vi "Write Elevator Direction.vi"(8 "error in (no error)":errorcluster, 10 "Elevator Direction":T1, 11 "Display Console in":refnum<class "Display Console.lvclass">) -> (0 "error out":errorcluster, 3 "Display Console out":refnum<class "Display Console.lvclass">)   [LabVIEW 2019, in "Display Console Actor.lvlib" / "Display Console.lvclass"]
uses:
  Display Console.lvclass
  Elevator Direction.ctl
  Display Console.lvclass/Display Console.ctl
  Abstract Display Console Actor/Abstract Display Console Actor/Abstract Display Console.lvclass
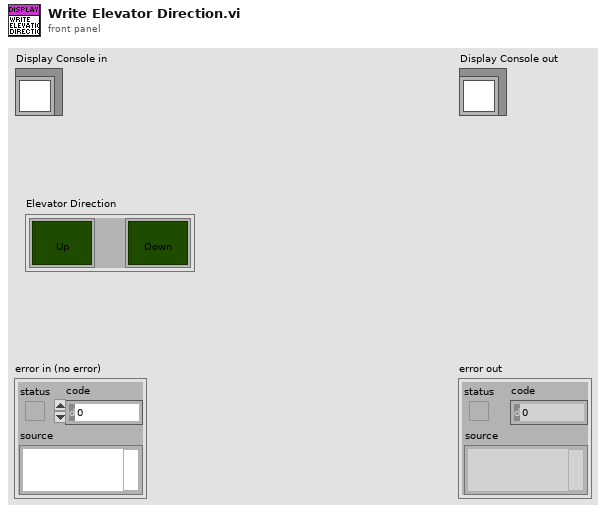
[diagram p1: front panel]
types:
  T1 = typedef "Display Console Actor.lvlib/Display Console.lvclass/Elevator Direction.ctl" = cluster{"Up":bool, "Down":bool}
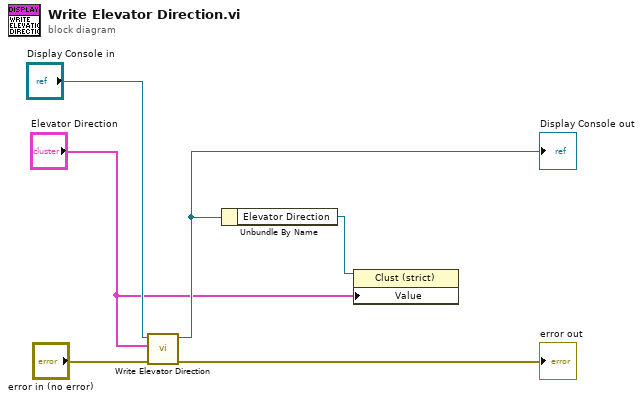
[diagram p0: block diagram]
diagram:
  n1 = call-parent "Write Elevator Direction.vi"("error in (no error)"="error in (no error)", "Elevator Direction"="Elevator Direction", "Abstract Display Console in"="Display Console in") -> ("error out"=→"error out":errorcluster, "Abstract Display Console out"=w3:refnum<class "Display Console.lvclass">)  [unwired: 7 in]
  "Display Console out" <- w3
  n2 = Unbundle By Name(w3) -> ("Elevator Direction"=w2:refnum<vi>)
  n3 = property class="Clust (strict)"(reference=w2, "Value"="Elevator Direction") -> ()  [unwired: 1 in, 2 out]
